vi "TemplateMethod.vi"(8 "ErrorIn":errorcluster, 9 "DummyIn":dbl, 11 "DotNETCamIn":refnum<class "DotNETCam.lvclass">) -> (0 "ErrorOut":errorcluster, 1 "DummyOut":dbl, 3 "DotNETCamOut":refnum<class "DotNETCam.lvclass">)   [LabVIEW 2021, in "DotNETCam.lvclass"]
uses:
  DotNETCam.lvclass
  C:/Localdata/Projects/TriekselSoft/TriekselsoftApplicationFramework/Source/.Externals/Library_YAF/YActor/YActor.lvclass
  DotNETCam_MsgCtrl.ctl
  .Externals/Library_YAF/YActor/YActor.lvclass/YActor.ctl
  .Externals/Library_YAF/YActor/ExeCmd_sync.vi
  .Externals/Library_YAF/YActor/private/SendCommand.vi
  .Externals/Library_YAF/YActor/private/WaitForReply.vi
  .Externals/Library_YAF/YActor/private/CreateLocalVI.vi
  .Externals/Library_YAF/YActor/private/ExeuteInlineVI.vi
  .Externals/Library_YAF/YActor/private/GetRemoteVIRef.vi
  .Externals/Library_YAF/YActor/private/GetNameOfVI.vi
  .Externals/Library_YAF/YActor/QuickCast.vi
  .Externals/Library_YAF/YActor/private/VINameProperty.vi
  .Externals/Library_YAF/YActor/private/MessageCounter.vi
  .Externals/Library_YAF/YActor/InlineReferencePool.vi
  .Externals/Library_YAF/YActor/private/ExecuteVI.vi
  .Externals/Library_YAF/YActor/YActor.lvclass
  C:/Localdata/Projects/TriekselSoft/TriekselsoftApplicationFramework/Source/.Externals/Library_YAF/YAFTAF/YAFTAF.lvclass
  C:/Localdata/Projects/TriekselSoft/TriekselsoftApplicationFramework/Source/.Externals/Interface_UserInterface_IFrontPanel/IFrontPanel/IFrontPanel.lvclass
  C:/Localdata/Projects/TriekselSoft/TriekselsoftApplicationFramework/Source/IInterface/IInterface.lvclass
  C:/Localdata/Projects/TriekselSoft/TriekselsoftApplicationFramework/Source/.Externals/Interface_Object_ICreateDestroy/ICreateDestroy/ICreateDestroy.lvclass
  C:/Localdata/Projects/TriekselSoft/TriekselsoftApplicationFramework/Source/.Externals/Interface_Object_IPersistentData/IPersistentData/IPersistentData.lvclass
  C:/Localdata/Projects/TriekselSoft/TriekselsoftApplicationFramework/Source/.Externals/Interface_TAF_ITAFObject/ITAFObject/ITAFObject.lvclass
  C:/Localdata/Projects/TriekselSoft/TriekselsoftApplicationFramework/Source/YAFTAFObjects/DotNETCam/DotNETCam.lvclass
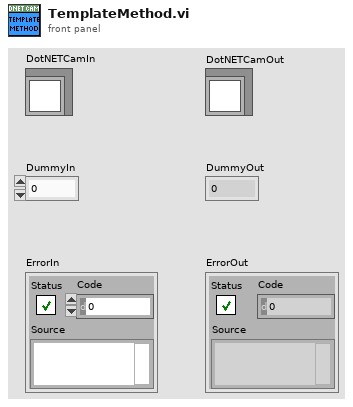
[diagram p1: front panel]
types:
  T1 = typedef "DotNETCam.lvclass/DotNETCam_MsgCtrl.ctl" = cluster{"TemplateCommand":cluster{"DummyIn":dbl, "DummyOut":dbl}}
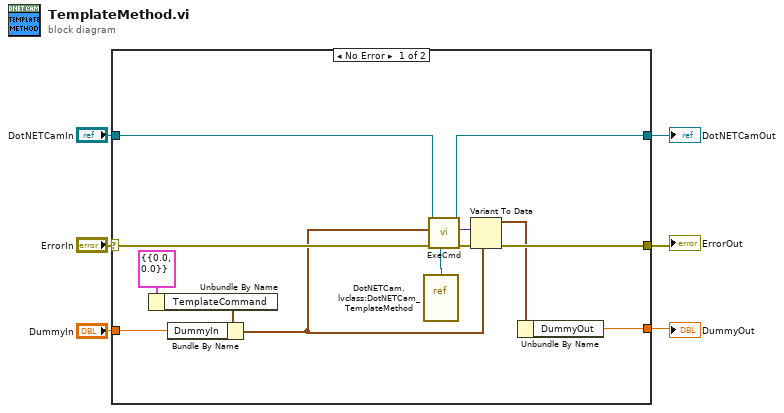
[diagram p0: block diagram]
diagram:
  n1 = case shown="No Error" "ErrorIn" {
    selector: "ErrorIn" -> [w19 w21]
    tunnel: [w17 w21] -> w5
    tunnel: [w7 w20] -> w3
    tunnel: "DotNETCamIn" -> [w8 w20]
    tunnel: "DummyIn" -> [w13 _]
    tunnel: [w9 _] -> w1
    frame No Error {
      n2 = Unbundle By Name(T1 {"TemplateCommand"={"DummyIn"=0.0, "DummyOut"=0.0}} ("MsgData")) -> ("TemplateCommand"=w14:cluster{"DummyIn":dbl, "DummyOut":dbl})
      n3 = Bundle By Name(cluster=w14, "DummyIn"=w13) -> (w11:cluster{"DummyIn":dbl, "DummyOut":dbl})
      n4 = vi-ref "DotNETCam.lvclass:DotNETCam_TemplateMethod.vi"() -> (w16:refnum<vi>)
      n5 = call-poly "ExeCmd.vi"("CmdVIRef"=w16, "ErrorIn"=w19, "CmdData"=w11, "YActorIn"=w8) -> ("ErrorOut"=w18:errorcluster, "ReplyData"=w12:variant, "YActorOut"=w7:refnum<class "DotNETCam.lvclass">)  [unwired: 5 in]
      n6 = Variant To Data(error in=w18, type=w11, Variant=w12) -> (data=w10:cluster{"DummyIn":dbl, "DummyOut":dbl}, error out=w17:errorcluster)
      n7 = Unbundle By Name(w10) -> ("DummyOut"=w9:dbl)
    }
    frame Error {
    }
  }
  "ErrorOut" <- w5
  "DotNETCamOut" <- w3
  "DummyOut" <- w1
